vi "getStyleByName.vi"(8 "error in (no error)":errorcluster, 10 "Style Name":string, 11 "Document in":refnum<class "Document.lvclass">) -> (0 "error out":errorcluster, 2 "Style":variant, 3 "Document out":refnum<class "Document.lvclass">)   [LabVIEW 2017, in "LabVIEW NPOI.lvlib" / "Document.lvclass"]
uses:
  Document.lvclass
  Document.lvclass/Document.ctl
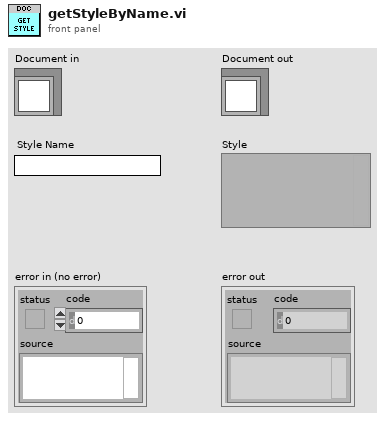
[diagram p1: front panel]
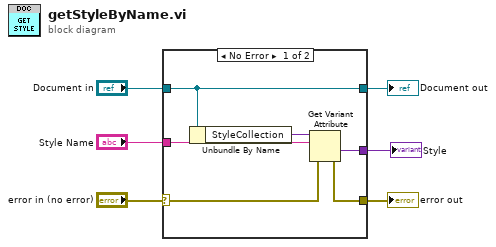
[diagram p0: block diagram]
diagram:
  n1 = case shown="No Error" "error in (no error)" {
    selector: "error in (no error)" -> [w8 w14]
    tunnel: [w7 w14] -> w5
    tunnel: [w12 w13] -> w3
    tunnel: "Document in" -> [w12 w13]
    tunnel: [w9 _] -> w2
    tunnel: "Style Name" -> [w10 _]
    frame No Error {
      n2 = Unbundle By Name(w12) -> ("StyleCollection"=w11:variant)
      n3 = Get Variant Attribute(Variant=w11, name=w10, error in=w8) -> (value=w9:variant, error out=w7:errorcluster)  [unwired: 1 in, 2 out]
    }
    frame Error {
    }
  }
  "error out" <- w5
  "Document out" <- w3
  "Style" <- w2
